vi "ws_get_target.vi"(7 "target_name":string) -> (0 "pool0":string, 1 "pool1":string, 2 "pool2":string, 3 "procs":u16, 4 "name":string, 6 "in_use":bool, 8 "user":string, 10 "Error?":bool, 11 "tag0":string, 12 "tag1":string, 13 "tag2":string, 14 "os":string, 15 "Error_info":string)   [LabVIEW 2011]
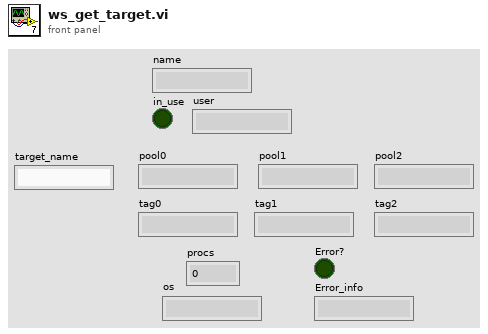
[diagram p1: front panel]
types:
  T1 = typedef "CommonTargetData.ctl" = cluster{"Name":string, "In Use?":bool, "User":string, " Pools":string[], "Tags":string[], "Procs":u16, "OS":string}
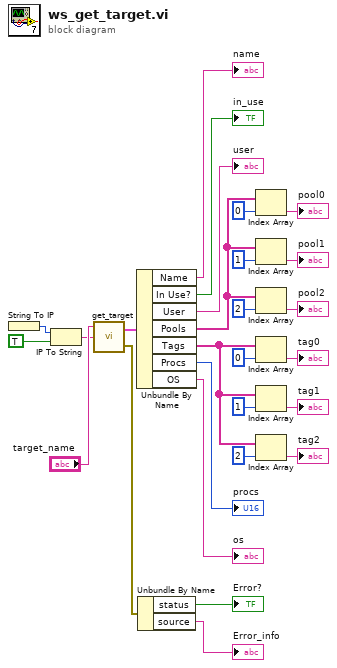
[diagram p0: block diagram]
diagram:
  n1 = String To IP() -> (0:w27:u32)  [unwired: 1 in]
  n2 = IP To String(1:TRUE ("dot notation? (F)"), 2:w27) -> (0:w22:string)
  n3 = call "get_target.vi"("Remote Server Address"=w22, "Name"="target_name") -> ("error out"=w20:errorcluster, "CommonTargetData"=w21:T1)  [unwired: 1 in]
  n4 = Unbundle By Name(w21) -> ("Name"=→"name":string, "In Use?"=→"in_use":bool, "User"=→"user":string, "Pools"=w14:string[], "Tags"=w4:string[], "Procs"=→"procs":u16, "OS"=→"os":string)
  n5 = Unbundle By Name(w20) -> ("status"=→"Error?":bool, "source"=→"Error_info":string)
  n6 = Index Array(array=w14, index=0) -> (element=→"pool0":string)
  n7 = Index Array(array=w14, index=1) -> (element=→"pool1":string)
  n8 = Index Array(array=w14, index=2) -> (element=→"pool2":string)
  n9 = Index Array(array=w4, index=0) -> (element=→"tag0":string)
  n10 = Index Array(array=w4, index=1) -> (element=→"tag1":string)
  n11 = Index Array(array=w4, index=2) -> (element=→"tag2":string)
